vi "Teleop.vi"(10 "Match Info":T2={"Autonomous Elapsed Seconds"=0.0, "TeleOp Elapsed Seconds"=0.0, "Disabled Elapsed Seconds"=0.0, "Visited Autonomous"=FALSE, "Visited TeleOp"=FALSE, "Visited Disabled"=FALSE, "Autonomous Settings"={"Autonomous Style"=enum."Independent", "VI Refnum"=refnum}}, 11 "Call Context":T3) -> ()   [LabVIEW 2012]
doc: "This VI is called for each TeleOp packet received from the DS where the robot is not disabled. It is often used to read from the joysticks and update I/O or to update setpoints for timed control loops. It should complete and return within 20 milliseconds or it may miss DS packets."
uses:
  <vilib>/Rock Robotics/WPI/DriverStation/WPI_DriverStationDerivedRobotMode.ctl
  <vilib>/Rock Robotics/WPI/DriverStation/WPI_DriverStationMatch Info.ctl
  <vilib>/Rock Robotics/WPI/Relay/WPI_RelayValue.ctl
  Robot Global Data.vi
  <vilib>/Rock Robotics/WPI/Joystick/WPI_JoystickGetSetRefNum.vi
panel:
  in  "Shoot":bool
  in  "FlipperUp":bool
  in  "Shoot":dbl=2.0
  in  "Retract":dbl=47.0
  in  "Down":dbl=150.0
  in  "Up":dbl=95.0
  in  "ShooterWheelB":dbl
  in  "ShooterWheelF":dbl
  in  "Dep Const":dbl=0.5
  in  "Roller Speed":dbl=0.75
  in  "RelayValue 2":T1
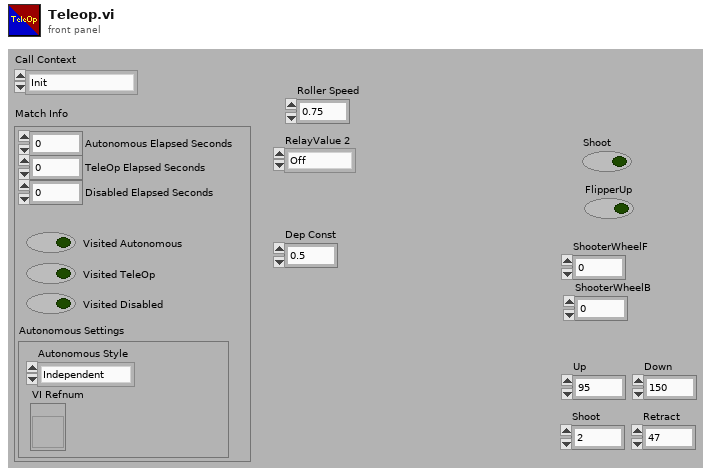
[diagram p1: front panel]
types:
  T1 = typedef "WPI_RelayValue.ctl" = enum16{"Off", "On", "Forward", "Reverse"}
  T2 = typedef "WPI_DriverStationMatch Info.ctl" = cluster{"Autonomous Elapsed Seconds":dbl, "TeleOp Elapsed Seconds":dbl, "Disabled Elapsed Seconds":dbl, "Visited Autonomous":bool, "Visited TeleOp":bool, "Visited Disabled":bool, "Autonomous Settings":cluster{"Autonomous Style":enum16{"Iterative", "Independent"}, "VI Refnum":refnum<vi>}}
  T3 = typedef "WPI_DriverStationDerivedRobotMode.ctl" = enum16{"Init", "Execute", "Stop"}
  T4 = typedef "WPI_ServoDeviceRef.ctl" = cluster{"DeviceStatus":errorcluster, "Digital Module":T5, "PWM Channel":T6, "DeadBand":T7}
  T5 = typedef "FPGA_TypedefDigitalModule.ctl" = enum16{"Digital Module 1", "Digital Module 2"}
  T6 = typedef "FPGA_DIOPWMChannel.ctl" = enum8{"PWM 1", "PWM 2", "PWM 3", "PWM 4", "PWM 5", "PWM 6", "PWM 7", "PWM 8", "PWM 9", "PWM 10", "Invalid"}
  T7 = typedef "WPI_PWMDeadband.ctl" = cluster{"Name":string, "maxPositivePwm":i32, "minPositivePwm":i32, "centerPwm":i32, "maxNegativePwm":i32, "minNegativePwm":i32, "angularRange":u16}
  T8 = typedef "WPI_MotorControlDeviceRef.ctl" = cluster{"DeviceStatus":errorcluster, "Type":enum16{"PWM", "CAN"}, "PWM":cluster{"Digital Module":T5, "PWM Channel":T6, "DeadBand":T7}, "CAN":cluster{"Device Number":u8, "Control Mode":T9, "Semaphore":T10, "Max Vout":dbl}, "Invert":bool, "TransformRef":T11, "InvTransformRef":T11}
  T9 = typedef "WPI_CANJaguar_ControlMode.ctl" = enum8{"Percent VBus", "Current", "Speed", "Position", "Voltage"}
  T10 = typedef "Semaphore RefNum" = refnum<k1>
  T11 = typedef "WPI_PWMTransform_ConPane.ctl" = refnum<vi>
  T12 = typedef "WPI_RelayDevRef.ctl" = cluster{"DevStatus":errorcluster, "Relay Channel":T13, "Digital Module":T5, "Relay Direction":T14}
  T13 = typedef "FPGA_DIORelayChannel.ctl" = enum8{"Relay 1", "Relay 2", "Relay 3", "Relay 4", "Relay 5", "Relay 6", "Relay 7", "Relay 8", "Invalid"}
  T14 = typedef "WPI_RelayDirection.ctl" = enum16{"Both directions", "Forward only", "Reverse only"}
  T15 = cluster{"Driver Station Digital Input (1-8)[0]":bool, "Driver Station Digital Input (1-8)[1]":bool, "Driver Station Digital Input (1-8)[2]":bool, "Driver Station Digital Input (1-8)[3]":bool, "Driver Station Digital Input (1-8)[4]":bool, "Driver Station Digital Input (1-8)[5]":bool, "Driver Station Digital Input (1-8)[6]":bool, "Driver Station Digital Input (1-8)[7]":bool, "Driver Station Digital Input (1-8)[8]":bool}
  T16 = cluster{"Right Servo High":dbl, "Right Servo Mid":dbl, "Right Servo Low":dbl, "Left Servo High":dbl, "Left Servo Mid":dbl, "Left Servo Low":dbl}
  T17 = typedef "WPI_JoystickDevRef.ctl" = cluster{"Device":T18}
  T18 = typedef "WPI_JoystickDeviceEnum.ctl" = enum16{"USB 1", "USB 2", "USB 3", "USB 4", "Kinect 1", "Kinect 2"}
  T19 = cluster{"axis 1 (x)":dbl, "axis 2 (y)":dbl, "axis 3 (throttle)":dbl, "axis 4":dbl, "axis 5":dbl, "axis 6":dbl}
  T20 = typedef "WPI_JoystickButtonState.ctl" = cluster{"Button 1":bool, "Button 2":bool, "Button 3":bool, "Button 4":bool, "Button 5":bool, "Button 6":bool, "Button 7":bool, "Button 8":bool, "Button 9":bool, "Button 10":bool, "Button 11":bool, "Button 12":bool}
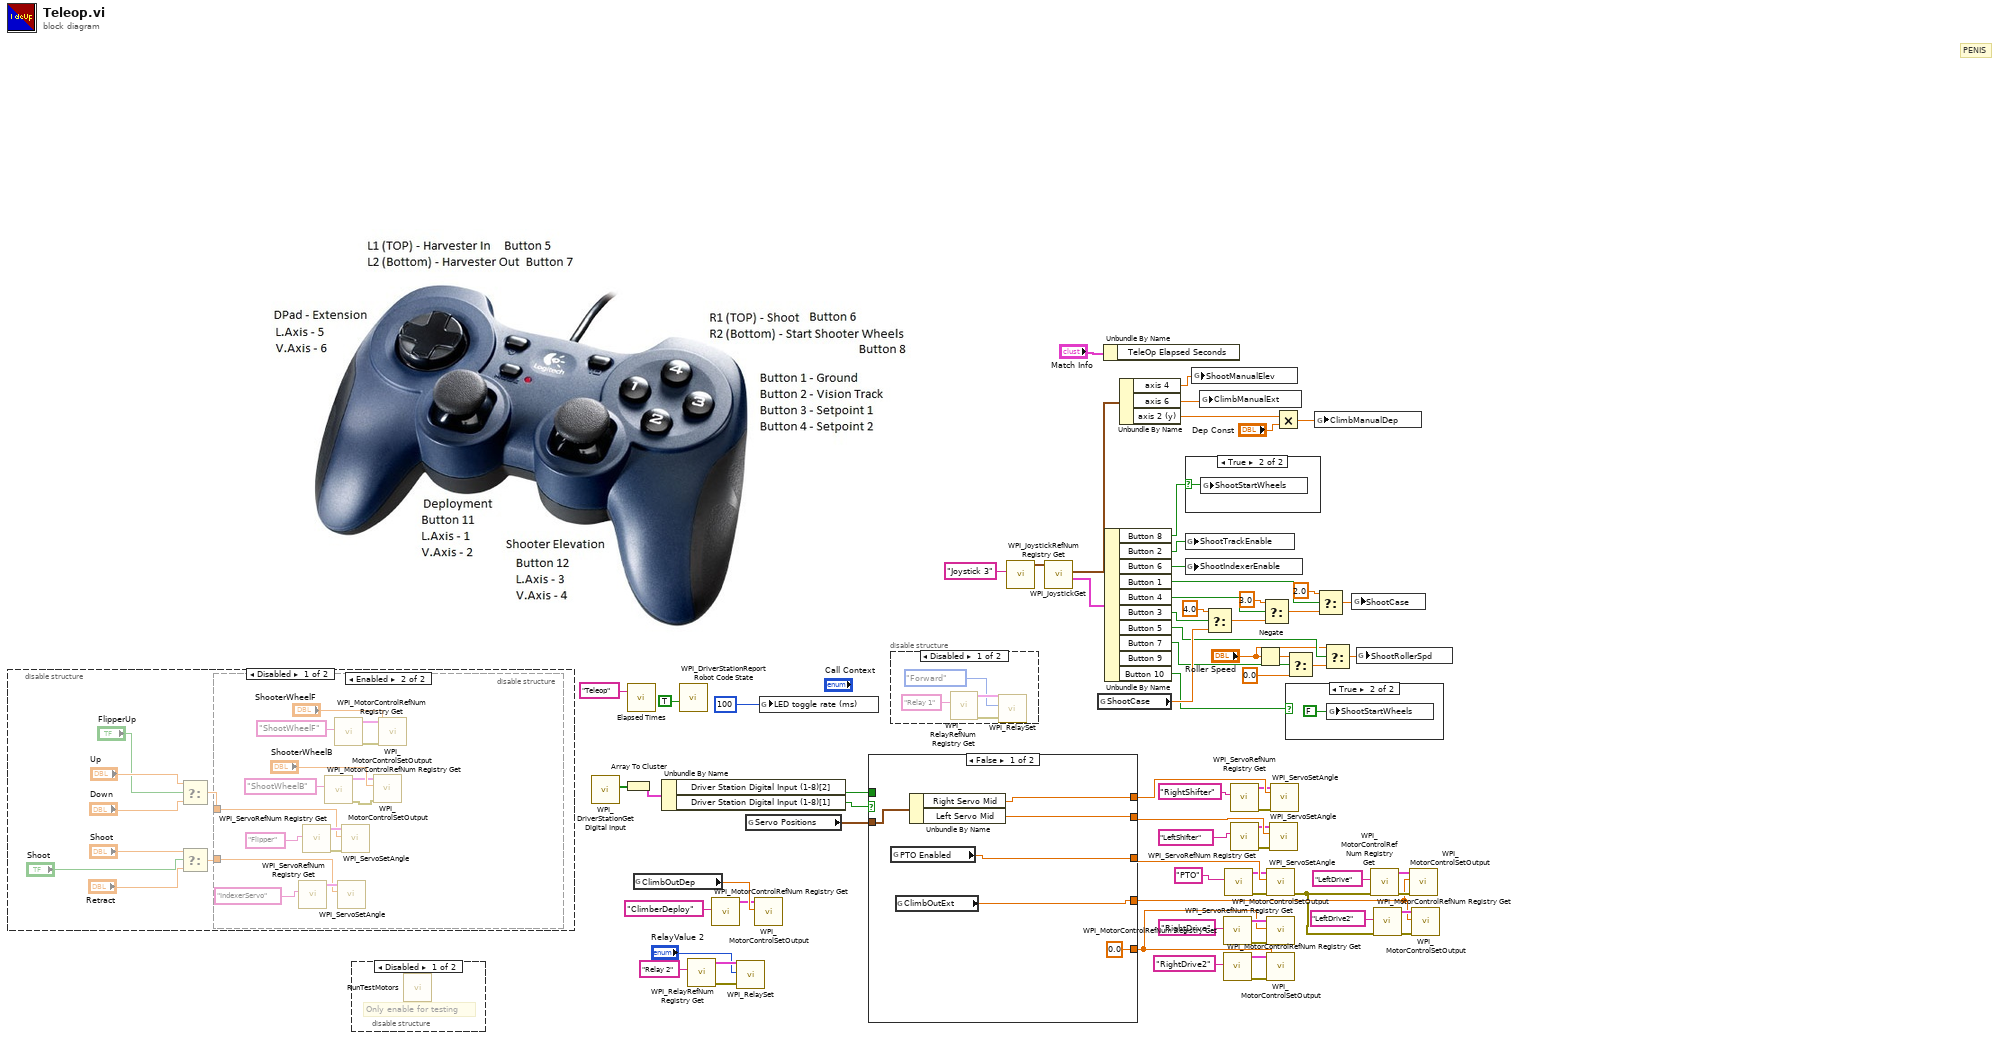
[diagram p0: block diagram]
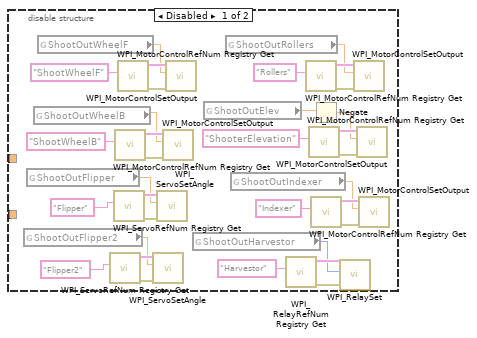
[diagram p2: hidden frame]
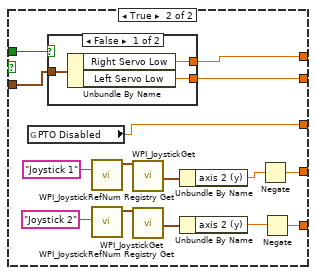
[diagram p6: hidden frame]
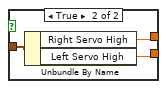
[diagram p7: hidden frame]
diagram:
  # "PENIS"
  n1 = disable-structure shown="Disabled" {
    frame Disabled {
      n2 = Select(t="Up", s="FlipperUp", f="Down") -> (s? t:f=w76:dbl)
      n3 = Select(t="Shoot", s="Shoot", f="Retract") -> (s? t:f=w75:dbl)
      n4 = disable-structure shown="Enabled" {
        disable-tunnel: w76 -> [_ w124]
        disable-tunnel: w75 -> [_ w123]
        frame Disabled {
          n5 = global read "Robot Global Data.vi" "ShootOutFlipper2"() -> (w86:dbl)
          n6 = global read "Robot Global Data.vi" "ShootOutFlipper"() -> (w87:dbl)
          n7 = global read "Robot Global Data.vi" "ShootOutWheelB"() -> (w94:dbl)
          n8 = global read "Robot Global Data.vi" "ShootOutWheelF"() -> (w99:dbl)
          n9 = call <vilib>:"WPI_ServoRefNum Registry Get.vi"("refnum name"="Flipper2") -> ("error out"=w90:errorcluster, "ServoDeviceRef"=w89:T4)  [unwired: 9 in]
          n10 = call <vilib>:"WPI_ServoRefNum Registry Get.vi"("refnum name"="Flipper") -> ("error out"=w91:errorcluster, "ServoDeviceRef"=w92:T4)  [unwired: 9 in]
          n11 = call <vilib>:"WPI_MotorControlRefNum Registry Get.vi"("refnum name"="ShootWheelB") -> ("error out"=w109:errorcluster, "MotorControlDevRef"=w110:T8)  [unwired: 9 in]
          n12 = call <vilib>:"WPI_MotorControlRefNum Registry Get.vi"("refnum name"="ShootWheelF") -> ("error out"=w114:errorcluster, "MotorControlDevRef"=w113:T8)  [unwired: 9 in]
          n13 = call <vilib>:"WPI_ServoSetAngle.vi"("error in (no error)"=w90, "Angle"=w86, "ServoDeviceRef"=w89) -> ()  [unwired: 7 in, 2 out]
          n14 = call <vilib>:"WPI_ServoSetAngle.vi"("error in (no error)"=w91, "Angle"=w87, "ServoDeviceRef"=w92) -> ()  [unwired: 7 in, 2 out]
          n15 = call <vilib>:"WPI_MotorControlSetOutput.vi"("error in (no error)"=w109, "Output"=w94, "MotorControlDevRef"=w110) -> ()  [unwired: 6 in, 3 out]
          n16 = call <vilib>:"WPI_MotorControlSetOutput.vi"("error in (no error)"=w114, "Output"=w99, "MotorControlDevRef"=w113) -> ()  [unwired: 6 in, 3 out]
          n17 = global read "Robot Global Data.vi" "ShootOutHarvestor"() -> (w82:T1)
          n18 = global read "Robot Global Data.vi" "ShootOutElev"() -> (w96:dbl)
          n19 = global read "Robot Global Data.vi" "ShootOutRollers"() -> (w97:dbl)
          n20 = global read "Robot Global Data.vi" "ShootOutIndexer"() -> (w98:dbl)
          n21 = call <vilib>:"WPI_RelayRefNum Registry Get.vi"("refnum name"="Harvestor") -> ("error out"=w85:errorcluster, "RelayDevRef"=w83:T12)  [unwired: 9 in]
          n22 = call <vilib>:"WPI_MotorControlRefNum Registry Get.vi"("refnum name"="Rollers") -> ("error out"=w106:errorcluster, "MotorControlDevRef"=w107:T8)  [unwired: 9 in]
          n23 = call <vilib>:"WPI_MotorControlRefNum Registry Get.vi"("refnum name"="ShooterElevation") -> ("error out"=w105:errorcluster, "MotorControlDevRef"=w104:T8)  [unwired: 9 in]
          n24 = Negate(x=w96) -> (-x=w95:dbl)
          n25 = call <vilib>:"WPI_MotorControlRefNum Registry Get.vi"("refnum name"="Indexer") -> ("error out"=w100:errorcluster, "MotorControlDevRef"=w101:T8)  [unwired: 9 in]
          n26 = call <vilib>:"WPI_RelaySet.vi"("error in (no error)"=w85, "RelayValue"=w82, "RelayDevRef"=w83) -> ()  [unwired: 7 in, 2 out]
          n27 = call <vilib>:"WPI_MotorControlSetOutput.vi"("error in (no error)"=w106, "Output"=w97, "MotorControlDevRef"=w107) -> ()  [unwired: 6 in, 3 out]
          n28 = call <vilib>:"WPI_MotorControlSetOutput.vi"("error in (no error)"=w105, "Output"=w95, "MotorControlDevRef"=w104) -> ()  [unwired: 6 in, 3 out]
          n29 = call <vilib>:"WPI_MotorControlSetOutput.vi"("error in (no error)"=w100, "Output"=w98, "MotorControlDevRef"=w101) -> ()  [unwired: 6 in, 3 out]
        }
        frame Enabled {
          n30 = call <vilib>:"WPI_ServoRefNum Registry Get.vi"("refnum name"="IndexerServo") -> ("ServoDeviceRef"=w128:T4)  [unwired: 9 in, 1 out]
          n31 = call <vilib>:"WPI_ServoRefNum Registry Get.vi"("refnum name"="Flipper") -> ("error out"=w127:errorcluster, "ServoDeviceRef"=w126:T4)  [unwired: 9 in]
          n32 = call <vilib>:"WPI_MotorControlRefNum Registry Get.vi"("refnum name"="ShootWheelB") -> ("error out"=w120:errorcluster, "MotorControlDevRef"=w121:T8)  [unwired: 9 in]
          n33 = call <vilib>:"WPI_MotorControlRefNum Registry Get.vi"("refnum name"="ShootWheelF") -> ("error out"=w116:errorcluster, "MotorControlDevRef"=w117:T8)  [unwired: 9 in]
          n34 = call <vilib>:"WPI_ServoSetAngle.vi"("Angle"=w123, "ServoDeviceRef"=w128) -> ()  [unwired: 8 in, 2 out]
          n35 = call <vilib>:"WPI_ServoSetAngle.vi"("error in (no error)"=w127, "Angle"=w124, "ServoDeviceRef"=w126) -> ()  [unwired: 7 in, 2 out]
          n36 = call <vilib>:"WPI_MotorControlSetOutput.vi"("error in (no error)"=w120, "Output"="ShooterWheelB", "MotorControlDevRef"=w121) -> ()  [unwired: 6 in, 3 out]
          n37 = call <vilib>:"WPI_MotorControlSetOutput.vi"("error in (no error)"=w116, "Output"="ShooterWheelF", "MotorControlDevRef"=w117) -> ()  [unwired: 6 in, 3 out]
        }
      }
    }
    frame Enabled {
    }
  }
  n38 = disable-structure shown="Disabled" {
    frame Disabled {
      # "Only enable for testing"
      n39 = call "RunTestMotors.vi"() -> ()  [unwired: 16 in]
    }
    frame Enabled {
    }
  }
  n40 = call <vilib>:"WPI_DriverStationGet Digital Input.vi"() -> ("Driver Station Digital Input (1-8)"=w33:bool[])  [unwired: 11 in]
  n41 = Array To Cluster(array=w33) -> (cluster=w32:T15)
  n42 = call "Elapsed Times.vi"("Call Name"="Teleop") -> ()  [unwired: 2 in, 1 out]
  n43 = global read "Robot Global Data.vi" "ClimbOutDep"() -> (w17:dbl)
  n44 = Unbundle By Name(w32) -> ("Driver Station Digital Input (1-8)[2]"=w31:bool, "Driver Station Digital Input (1-8)[1]"=w23:bool)
  n45 = call <vilib>:"WPI_DriverStationReport Robot Code State.vi"("TeleOp"=TRUE ("Autonomous")) -> ()  [unwired: 10 in, 1 out]
  n46 = call <vilib>:"WPI_RelayRefNum Registry Get.vi"("refnum name"="Relay 2") -> ("error out"=w2:errorcluster, "RelayDevRef"=w4:T12)  [unwired: 9 in]
  n47 = call <vilib>:"WPI_MotorControlRefNum Registry Get.vi"("refnum name"="ClimberDeploy") -> ("MotorControlDevRef"=w15:T8)  [unwired: 9 in, 1 out]
  n48 = call <vilib>:"WPI_RelaySet.vi"("error in (no error)"=w2, "RelayValue"="RelayValue 2", "RelayDevRef"=w4) -> ()  [unwired: 7 in, 2 out]
  n49 = global read "Robot Global Data.vi" "Servo Positions"() -> (w30:T16)
  n50 = call <vilib>:"WPI_MotorControlSetOutput.vi"("Output"=w17, "MotorControlDevRef"=w15) -> ()  [unwired: 7 in, 3 out]
  n51 = global write "Robot Global Data.vi" "LED toggle rate (ms)"(u32 100 ("LED ms toggle rate")) -> ()
  n52 = case shown="False" w23 {
    tunnel: w31 -> [_ w150]
    tunnel: w30 -> [w135 w149]
    tunnel: [w134 w148] -> w29
    tunnel: [w133 w147] -> w28
    tunnel: [w132 w146] -> w20
    tunnel: [w130 w137] -> w19
    tunnel: [0.0 w136] -> w18
    frame False {
      n53 = global read "Robot Global Data.vi" "PTO Enabled"() -> (w132:dbl)
      n54 = global read "Robot Global Data.vi" "ClimbOutExt"() -> (w130:dbl)
      n55 = Unbundle By Name(w135) -> ("Right Servo Mid"=w134:dbl, "Left Servo Mid"=w133:dbl)
    }
    frame True {
      n56 = global read "Robot Global Data.vi" "PTO Disabled"() -> (w146:dbl)
      n57 = case shown="False" w150 {
        tunnel: w149 -> [w153 w156]
        tunnel: [w152 w155] -> w148
        tunnel: [w151 w154] -> w147
        frame False {
          n58 = Unbundle By Name(w153) -> ("Right Servo Low"=w152:dbl, "Left Servo Low"=w151:dbl)
        }
        frame True {
          n59 = Unbundle By Name(w156) -> ("Right Servo High"=w155:dbl, "Left Servo High"=w154:dbl)
        }
      }
      n60 = call <vilib>:"WPI_JoystickRefNum Registry Get.vi"("refnum name"="Joystick 1") -> ("JoystickDevRef"=w138:T17)  [unwired: 1 in, 9 out]
      n61 = call <vilib>:"WPI_JoystickRefNum Registry Get.vi"("refnum name"="Joystick 2") -> ("JoystickDevRef"=w144:T17)  [unwired: 1 in, 9 out]
      n62 = call <vilib>:"WPI_JoystickGet.vi"("JoystickDevRef"=w138) -> ("Axes"=w141:T19)  [unwired: 1 in, 5 out]
      n63 = call <vilib>:"WPI_JoystickGet.vi"("JoystickDevRef"=w144) -> ("Axes"=w145:T19)  [unwired: 1 in, 5 out]
      n64 = Unbundle By Name(w141) -> ("axis 2 (y)"=w140:dbl)
      n65 = Unbundle By Name(w145) -> ("axis 2 (y)"=w142:dbl)
      n66 = Negate(x=w140) -> (-x=w137:dbl)
      n67 = Negate(x=w142) -> (-x=w136:dbl)
    }
  }
  n68 = disable-structure shown="Disabled" {
    frame Disabled {
      n69 = call <vilib>:"WPI_RelayRefNum Registry Get.vi"("refnum name"="Relay 1") -> ("error out"=w158:errorcluster, "RelayDevRef"=w160:T12)  [unwired: 9 in]
      n70 = call <vilib>:"WPI_RelaySet.vi"("error in (no error)"=w158, "RelayValue"=WPI_RelayValue."Forward", "RelayDevRef"=w160) -> ()  [unwired: 7 in, 2 out]
    }
    frame Enabled {
    }
  }
  n71 = call <vilib>:"WPI_JoystickRefNum Registry Get.vi"("refnum name"="Joystick 3") -> ("JoystickDevRef"=w70:T17)  [unwired: 9 in, 1 out]
  n72 = call <vilib>:"WPI_JoystickGet.vi"("JoystickDevRef"=w70) -> ("Buttons"=w68:T20, "Axes"=w67:T19)  [unwired: 4 in, 1 out]
  n73 = global read "Robot Global Data.vi" "ShootCase"() -> (w55:dbl)
  n74 = Unbundle By Name("Match Info") -> ()  [unwired: 1 out]
  n75 = Unbundle By Name(w68) -> ("Button 8"=w48:bool, "Button 2"=w65:bool, "Button 6"=w66:bool, "Button 1"=w63:bool, "Button 4"=w61:bool, "Button 3"=w60:bool, "Button 5"=w51:bool, "Button 7"=w53:bool, "Button 10"=w47:bool)  [unwired: 1 out]
  n76 = Unbundle By Name(w67) -> ("axis 4"=w64:dbl, "axis 6"=w1:dbl, "axis 2 (y)"=w7:dbl)
  n77 = case shown="True" w48 {
    selector: w48 -> [_ w161]
    frame False {
    }
    frame True {
      n78 = global write "Robot Global Data.vi" "ShootStartWheels"(w161) -> ()
    }
  }
  n79 = global write "Robot Global Data.vi" "ShootTrackEnable"(w65) -> ()
  n80 = global write "Robot Global Data.vi" "ShootIndexerEnable"(w66) -> ()
  n81 = global write "Robot Global Data.vi" "ShootManualElev"(w64) -> ()
  n82 = global write "Robot Global Data.vi" "ClimbManualExt"(w1) -> ()
  n83 = Select(t=4.0, s=w60, f=w55) -> (s? t:f=w59:dbl)
  n84 = call <vilib>:"WPI_MotorControlRefNum Registry Get.vi"("refnum name"="RightDrive") -> ("error out"=w43:errorcluster, "MotorControlDevRef"=w45:T8)  [unwired: 9 in]
  n85 = call <vilib>:"WPI_MotorControlRefNum Registry Get.vi"("refnum name"="RightDrive2") -> ("error out"=w36:errorcluster, "MotorControlDevRef"=w34:T8)  [unwired: 9 in]
  n86 = call <vilib>:"WPI_ServoRefNum Registry Get.vi"("refnum name"="PTO") -> ("error out"=w13:errorcluster, "ServoDeviceRef"=w14:T4)  [unwired: 9 in]
  n87 = call <vilib>:"WPI_ServoRefNum Registry Get.vi"("refnum name"="RightShifter") -> ("error out"=w24:errorcluster, "ServoDeviceRef"=w25:T4)  [unwired: 9 in]
  n88 = call <vilib>:"WPI_ServoRefNum Registry Get.vi"("refnum name"="LeftShifter") -> ("error out"=w26:errorcluster, "ServoDeviceRef"=w27:T4)  [unwired: 9 in]
  n89 = Negate(x="Roller Speed") -> (-x=w11:dbl)
  n90 = Select(t=3.0, s=w61, f=w59) -> (s? t:f=w57:dbl)
  n91 = call <vilib>:"WPI_ServoSetAngle.vi"("error in (no error)"=w13, "Angle"=w20, "ServoDeviceRef"=w14) -> ("error out"=w6:errorcluster)  [unwired: 7 in, 1 out]
  n92 = call <vilib>:"WPI_MotorControlSetOutput.vi"("error in (no error)"=w43, "Output"=w18, "MotorControlDevRef"=w45) -> ()  [unwired: 6 in, 3 out]
  n93 = call <vilib>:"WPI_MotorControlSetOutput.vi"("error in (no error)"=w36, "Output"=w18, "MotorControlDevRef"=w34) -> ()  [unwired: 6 in, 3 out]
  n94 = call <vilib>:"WPI_ServoSetAngle.vi"("error in (no error)"=w26, "Angle"=w28, "ServoDeviceRef"=w27) -> ()  [unwired: 7 in, 2 out]
  n95 = call <vilib>:"WPI_ServoSetAngle.vi"("error in (no error)"=w24, "Angle"=w29, "ServoDeviceRef"=w25) -> ()  [unwired: 7 in, 2 out]
  n96 = Multiply(x=w7, y="Dep Const") -> (x*y=w9:dbl)
  n97 = case shown="True" w47 {
    frame False {
    }
    frame True {
      n98 = global write "Robot Global Data.vi" "ShootStartWheels"(FALSE ("ShootStartWheels")) -> ()
    }
  }
  n99 = Select(t=w11, s=w53, f=0.0) -> (s? t:f=w52:dbl)
  n100 = global write "Robot Global Data.vi" "ClimbManualDep"(w9) -> ()
  n101 = Select(t=2.0, s=w63, f=w57) -> (s? t:f=w54:dbl)
  n102 = Select(t="Roller Speed", s=w51, f=w52) -> (s? t:f=w49:dbl)
  n103 = global write "Robot Global Data.vi" "ShootCase"(w54) -> ()
  n104 = global write "Robot Global Data.vi" "ShootRollerSpd"(w49) -> ()
  n105 = call <vilib>:"WPI_MotorControlRefNum Registry Get.vi"("error in (no error)"=w6, "refnum name"="LeftDrive") -> ("error out"=w38:errorcluster, "MotorControlDevRef"=w41:T8)  [unwired: 8 in]
  n106 = call <vilib>:"WPI_MotorControlRefNum Registry Get.vi"("error in (no error)"=w6, "refnum name"="LeftDrive2") -> ("error out"=w37:errorcluster, "MotorControlDevRef"=w39:T8)  [unwired: 8 in]
  n107 = call <vilib>:"WPI_MotorControlSetOutput.vi"("error in (no error)"=w38, "Output"=w19, "MotorControlDevRef"=w41) -> ()  [unwired: 6 in, 3 out]
  n108 = call <vilib>:"WPI_MotorControlSetOutput.vi"("error in (no error)"=w37, "Output"=w19, "MotorControlDevRef"=w39) -> ()  [unwired: 6 in, 3 out]
